vi "init.vi"(8 "error in (no error)":errorcluster, 11 "Compensator in":refnum<class "SystemController.lvclass">) -> (0 "error out":errorcluster, 3 "Compensator out":refnum<class "SystemController.lvclass">)   [LabVIEW 2013, in "SystemController.lvclass"]
uses:
  SystemController/SystemController.lvclass
  Configuration/System Controller.ctl
  Configuration/PIDGains.ctl
  SystemController/SystemController.lvclass/SystemController.ctl
  ConfigurationThisComponent/ConfigurationThisComponent.lvclass
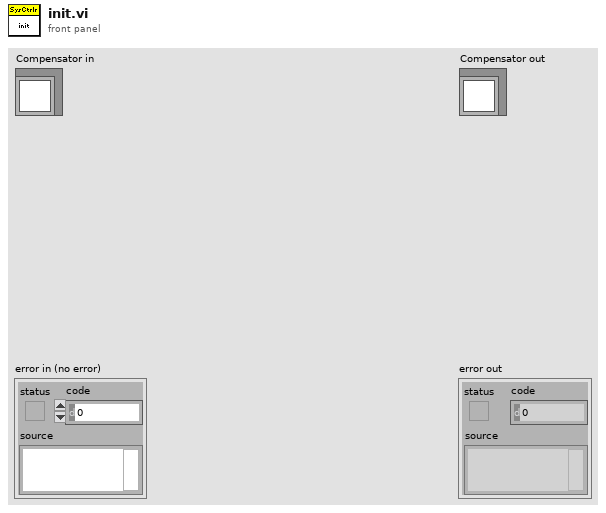
[diagram p1: front panel]
types:
  T1 = typedef "System Controller.ctl" = cluster{"PID Gains":T2, "Force Error In Range Limit":dbl[unit]}
  T2 = typedef "PIDGains.ctl" = cluster{"Proportional Gain (Kc)":dbl, "Integral Time (Ti, min)":dbl, "Derivative Time (Td, min)":dbl}
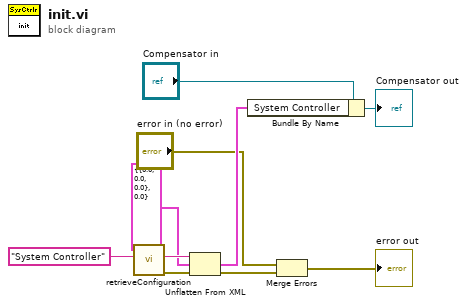
[diagram p0: block diagram]
diagram:
  n1 = call "retrieveConfiguration.vi"("configName"="System Controller") -> ("error out"=w7:errorcluster, "xmlConfig"=w6:string)  [unwired: 8 in, 1 out]
  n2 = Unflatten From XML(xml string=w6, type=T1 {"PID Gains"={"Proportional Gain (Kc)"=0.0, "Integral Time (Ti, min)"=0.0, "Derivative Time (Td, min)"=0.0}, "Force Error In Range Limit"=0.0} ("Compensator"), error in (no error)=w7) -> (value=w10:T1, error out=w9:errorcluster)
  n3 = Bundle By Name(cluster="Compensator in", "System Controller"=w10) -> (→"Compensator out":refnum<class "SystemController.lvclass">)
  n4 = Merge Errors("error in (no error)", w9) -> (→"error out":errorcluster)
